vi "Computer current I SubVI).vi"(6 "V":dbl, 9 "G":dbl, 10 "T":dbl, 11 "I_1":dbl) -> (1 "I":dbl, 2 "I_0":dbl, 3 "I_rs":dbl, 4 "I_ph":dbl, 5 "I_sh":dbl)   [LabVIEW 2024]
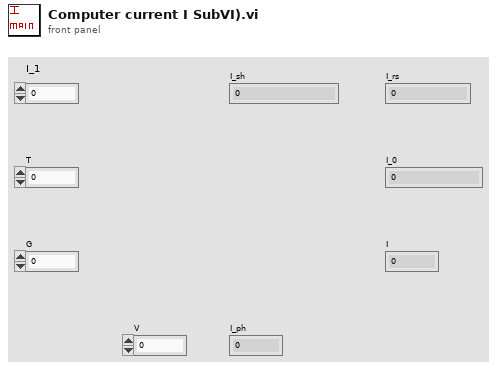
[diagram p1: front panel]
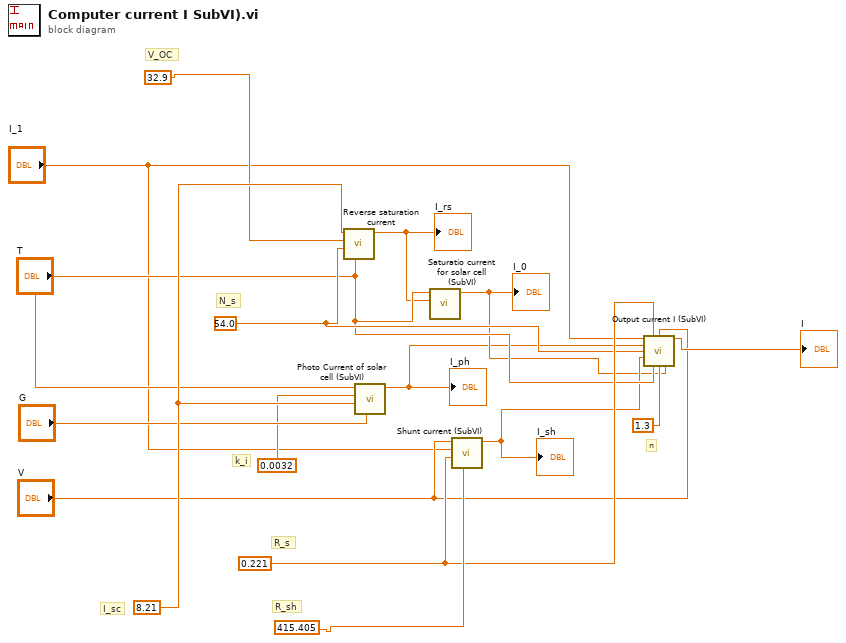
[diagram p0: block diagram]
diagram:
  w15 = 0.221 ("R_s")
  w14 = 54.0 ("N_s")
  w13 = 8.21 ("I_sc")
  # "n"
  # "R_sh"
  # "R_s"
  # "k_i"
  # "N_s"
  # "I_sc"
  # "V_OC"
  n1 = call "Reverse saturation current.vi"("T"="T", "N_s"=w14, "V_OC"=32.9, "I_sc"=w13) -> ("I_rs"=w4:dbl)  [unwired: 7 in]
  "I_rs" <- w4
  n2 = call "Photo Current of solar cell (SubVI).vi"("G"="G", "I_sc"=w13, "k_i"=0.0032, "T"="T") -> ("I_ph"=w5:dbl)  [unwired: 7 in]
  "I_ph" <- w5
  n3 = call "Saturatio current for solar cell (SubVI).vi"("I_rs"=w4, "T"="T") -> ("I_0"=w6:dbl)  [unwired: 9 in]
  "I_0" <- w6
  n4 = call "Shunt current (SubVI).vi"("R_sh"=415.405, "R_s"=w15, "I"="I_1", "V"="V") -> ("I_sh"=w7:dbl)  [unwired: 7 in]
  "I_sh" <- w7
  n5 = call "Output current I (SubVI).vi"("I_1"="I_1", "R_s"=w15, "V"="V", "I_ph"=w5, "N_s"=w14, "I_sh"=w7, "T"="T", "n"=1.3, "I_0"=w6) -> ("I"=→"I":dbl)  [unwired: 6 in]
